vi "Run Main.vi"(8 "error in":errorcluster) -> (0 "error out":errorcluster)   [LabVIEW 2020, in "GUI.lvlib"]
uses:
  GUI.lvlib
  Shared Ressources/gamepad-direction-enum.ctl
  Shared Ressources/Controller-button-pressed-enum.ctl
  SubVIs and TypeDefs/Runtime Data.ctl
  SubVIs and TypeDefs/Eventing/Event FGV Actions.ctl
  Shared Ressources/gui-data-to-display-cluster.ctl
  Shared Ressources/latest-controller-inputs.ctl
  Manager/Manager.lvlib
panel:
  out "time":string
  out "latest button pressed enum":T1
  out "latest gamepad direction":T2
  out "information":string
  out "Direction":T3
  out "buttons":T4
  # "Gamepad Controller Interface"
  # "Demo Version - Developped by Antoine BENOIT"
  # "Latest keys"
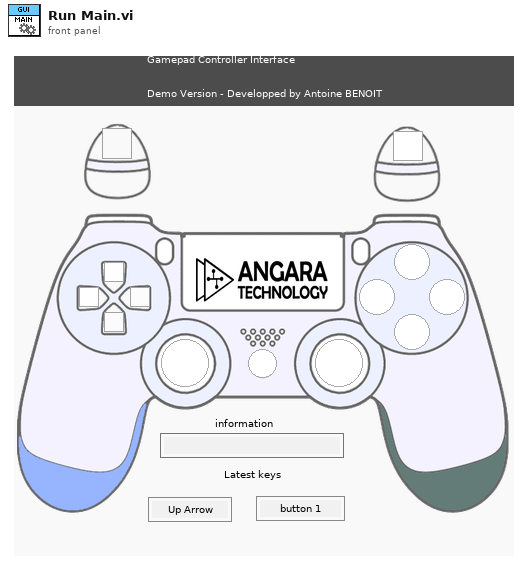
[diagram p1: front panel]
types:
  T1 = typedef "Controller-button-pressed-enum.ctl" = enum16{"button 1", "button 2", "button 3", "button 4", "button 5", "button 6", "button 7", "button 8", "button 9", "button 10", "button 11", "button 12", "button 13", "button 14"}
  T2 = typedef "gamepad-direction-enum.ctl" = enum16{"Up Arrow", "Right Arrow", "Down Arrow", "Left Arrow"}
  T3 = cluster{"up":bool, "right":bool, "down":bool, "left":bool}
  T4 = cluster{"Boolean 2":bool, "Boolean 4":bool, "Boolean 3":bool, "Boolean":bool, "Boolean 17":bool, "Boolean 18":bool, "Boolean 5":bool, "Boolean 6":bool, "Boolean 15":bool, "Boolean 14":bool, "Boolean 10":bool, "Boolean 9":bool, "Boolean 12":bool, "Boolean 16":bool}
  T5 = typedef "GUI.lvlib/Event FGV Actions.ctl" = enum16{"Get", "Create", "Destroy"}
  T6 = typedef "GUI.lvlib/Runtime Data.ctl" = cluster{"sn":string}
  T7 = typedef "gui-data-to-display-cluster.ctl" = cluster{"latest controller inputs":T8, "information":string}
  T8 = typedef "latest-controller-inputs.ctl" = cluster{"Controller button pressed enum":T1, "gamepad direction":T2}
  T9 = cluster{"[0]":bool, "[1]":bool, "[2]":bool, "[3]":bool, "[4]":bool, "[5]":bool, "[6]":bool, "[7]":bool, "[8]":bool, "[9]":bool, "[10]":bool, "[11]":bool, "[12]":bool, "[13]":bool}
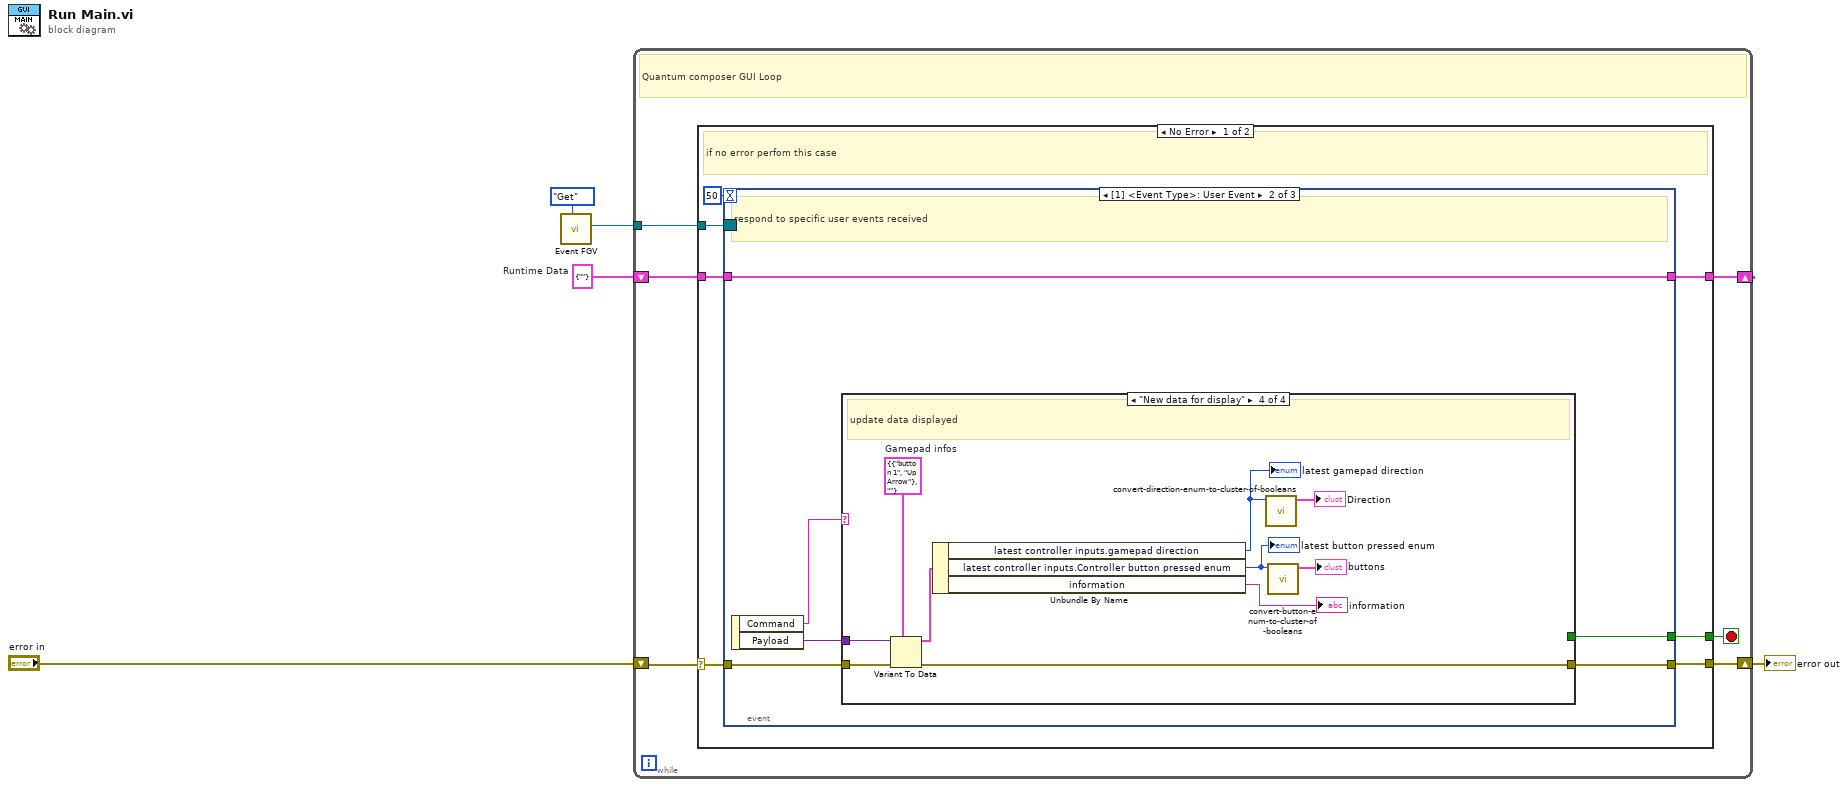
[diagram p0: block diagram]
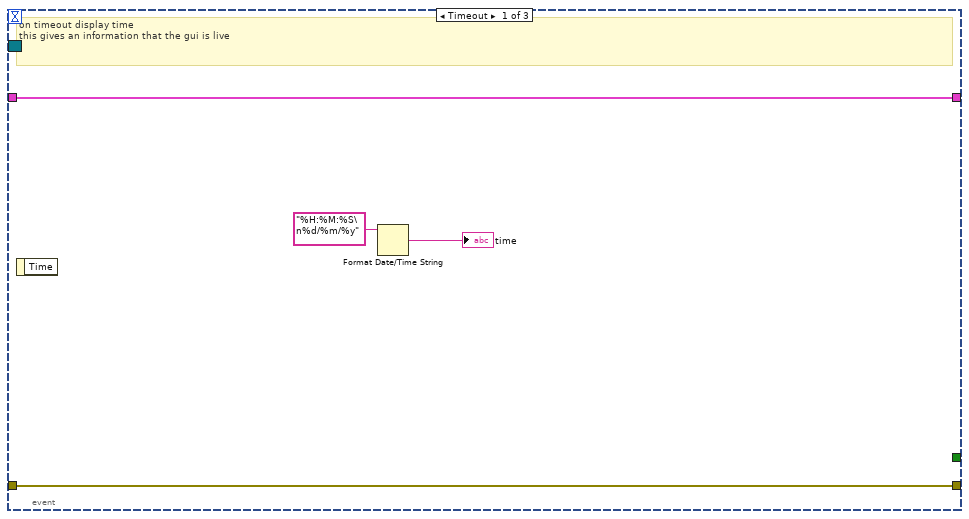
[diagram p2: hidden frame]
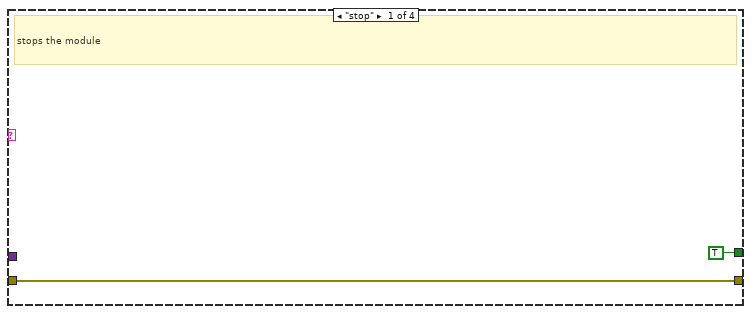
[diagram p3: hidden frame]
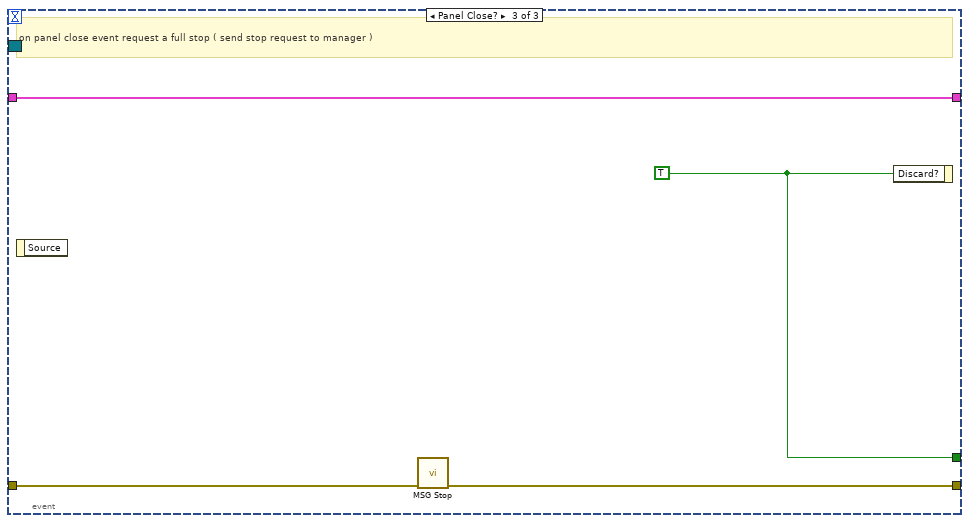
[diagram p6: hidden frame]
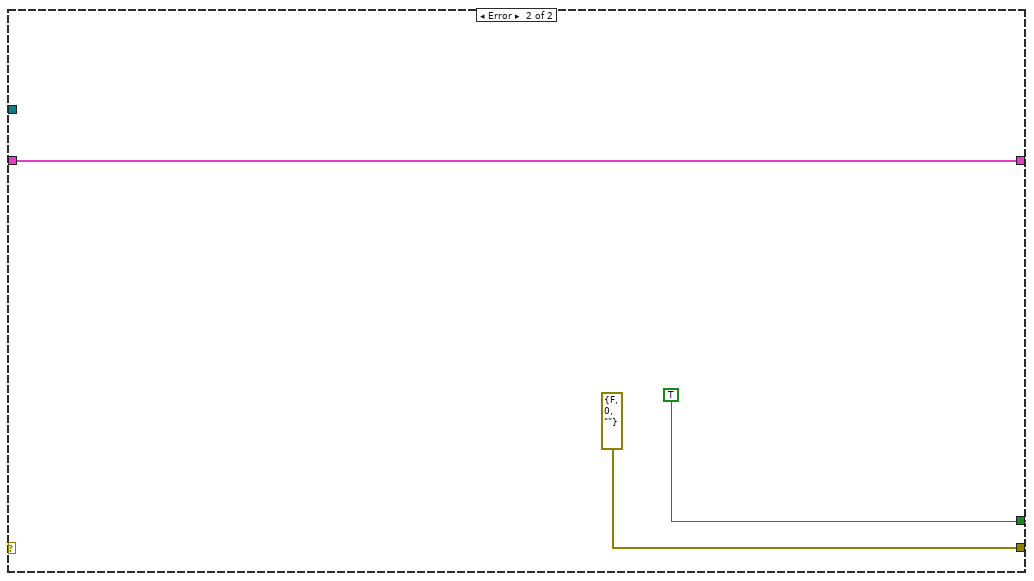
[diagram p7: hidden frame]
diagram:
  w3 = T6 {"sn"=""}  # Runtime Data
  n1 = call "Event FGV.vi"("Event FGV Actions"=Event_FGV_Actions."Get") -> ("Event Registration Refnum"=w4:refnum<event-registration>)  [unwired: 8 in, 2 out]
  n2 = while {
    tunnel: w4 -> [w9]
    shift-right: [w8] -> _
    shift-left: w3 -> [w7]
    shift-right: [w6] -> w2
    shift-left: "error in" -> [w10]
    stop <- w11 stop-if-true
    # "Quantum composer GUI Loop"
    n3 = case shown="No Error" w10 {
      selector: w10 -> [w14 _]
      tunnel: [w18 TRUE] -> w11
      tunnel: w9 -> [w17 _]
      tunnel: [w16 w48] -> w8
      tunnel: w7 -> [w15 w48]
      tunnel: [w13 errorcluster {"status"=FALSE, "code"=0, "source"=""} ("error out")] -> w6
      frame No Error {
        # "if no error perfom this case"
        n4 = event shown="[1] <Event Type>: User Event" {
          selector: w17 -> [_ _ _]
          dyn-events: _ -> [_ _ _]
          timeout: 50 -> [_ _ _]
          tunnel: [_ w23 w46] -> w18
          tunnel: [w22 w24 w45] -> w16
          tunnel: w15 -> [w22 w24 w45]
          tunnel: w14 -> [w21 w26 w44]
          tunnel: [w21 w25 w43] -> w13
          event Timeout {
            # "on timeout display time\nthis gives an information that the gui is live"
            n5 = event-data() -> ()  [unwired: 1 in, 1 out]
            n6 = Format Date/Time String(time format string (%c)="%H:%M:%S\n%d/%m/%y") -> (date/time string=→"time":string)  [unwired: 2 in]
          }
          event User Event {
            # "respond to specific user events received"
            n7 = event-data() -> ("Command"=w28:string, "Payload"=w27:variant)  [unwired: 1 in]
            n8 = case shown="\"New data for display\"" w28 {
              tunnel: w27 -> [_ _ _ w40]
              tunnel: w26 -> [w30 w31 w32 w42]
              tunnel: [w30 w31 w32 w41] -> w25
              tunnel: [TRUE _ _ _] -> w23
              frame "stop" {
                # "stops the module"
              }
              frame Default {
                # "default case should not happen"
              }
              frame "init" {
                # "init case ( use if need be )"
              }
              frame "New data for display" {
                w39 = T7 {"latest controller inputs"={"Controller button pressed enum"=enum."button 1", "gamepad direction"=enum."Up Arrow"}, "information"=""}  # Gamepad infos
                # "update data displayed"
                n9 = Variant To Data(error in=w42, type=w39, Variant=w40) -> (data=w38:T7, error out=w41:errorcluster)
                n10 = Unbundle By Name(w38) -> ("latest controller inputs.gamepad direction"=w37:T2, "latest controller inputs.Controller button pressed enum"=w35:T1, "information"=→"information":string)
                "latest gamepad direction" <- w37
                "latest button pressed enum" <- w35
                n11 = call "convert-direction-enum-to-cluster-of-booleans.vi"("gamepad direction"=w37) -> ("Direction"=→"Direction":T3)  [unwired: 10 in]
                n12 = call "convert-button-enum-to-cluster-of-booleans.vi"("Controller button pressed enum"=w35) -> ("Cluster"=→"buttons":T9)  [unwired: 10 in]
              }
            }
          }
          event Panel Close? {
            w46 = TRUE ("Discard?")
            # "on panel close event request a full stop ( send stop request to manager )"
            n13 = event-data() -> ()  [unwired: 1 in, 1 out]
            n14 = call "MSG Stop.vi"("error in"=w44) -> ("error out"=w43:errorcluster)  [unwired: 10 in]
            n15 = event-data("Discard?"=w46) -> ()  [unwired: 1 in, 1 out]
          }
        }
      }
      frame Error {
      }
    }
  }
  "error out" <- w2
